vi "Clock Example.vi"() -> ()   [LabVIEW 2015]
uses:
  Forms/Rectangle/Rectangle.lvclass
  Image Editor Handler/Image Editor Handler.lvclass
  Forms/Shape/Shape.lvclass/Shape.ctl
  Forms/Rectangle/Rectangle.lvclass/Rectangle.ctl
  Forms/Shape/Write Color.vi
  Forms/Rectangle/Write Filled.vi
  Forms/Shape/Write Movable.vi
  Forms/Shape/Write Selectable.vi
  Forms/Shape/Shape.lvclass
  Forms/Link/Link.lvclass
panel:
  in  "2D Picture":picture
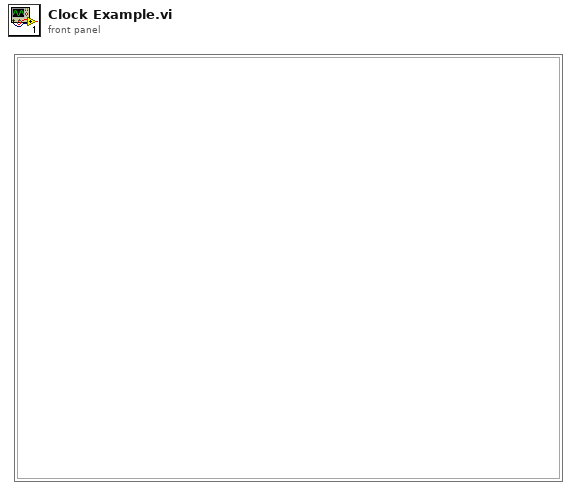
[diagram p1: front panel]
types:
  T1 = cluster{"Width":u16, "Style":enum32{"Solid", "Dash", "Dot", "DashDot", "DashDotDot"}}
  T2 = typedef "LVBoundsTypeDef.ctl" = cluster{"Width":u32, "Height":u32}
  T3 = cluster{"Rayon H":dbl, "Rayon M":dbl, "Rayon S":dbl}
  T4 = typedef "LVDateTimeRec.ctl" = cluster{"fractional second":dbl, "second":i32, "minute":i32, "hour":i32, "day of month":i32, "month":i32, "year":i32, "day of week":i32, "day of year":i32, "DST":i32}
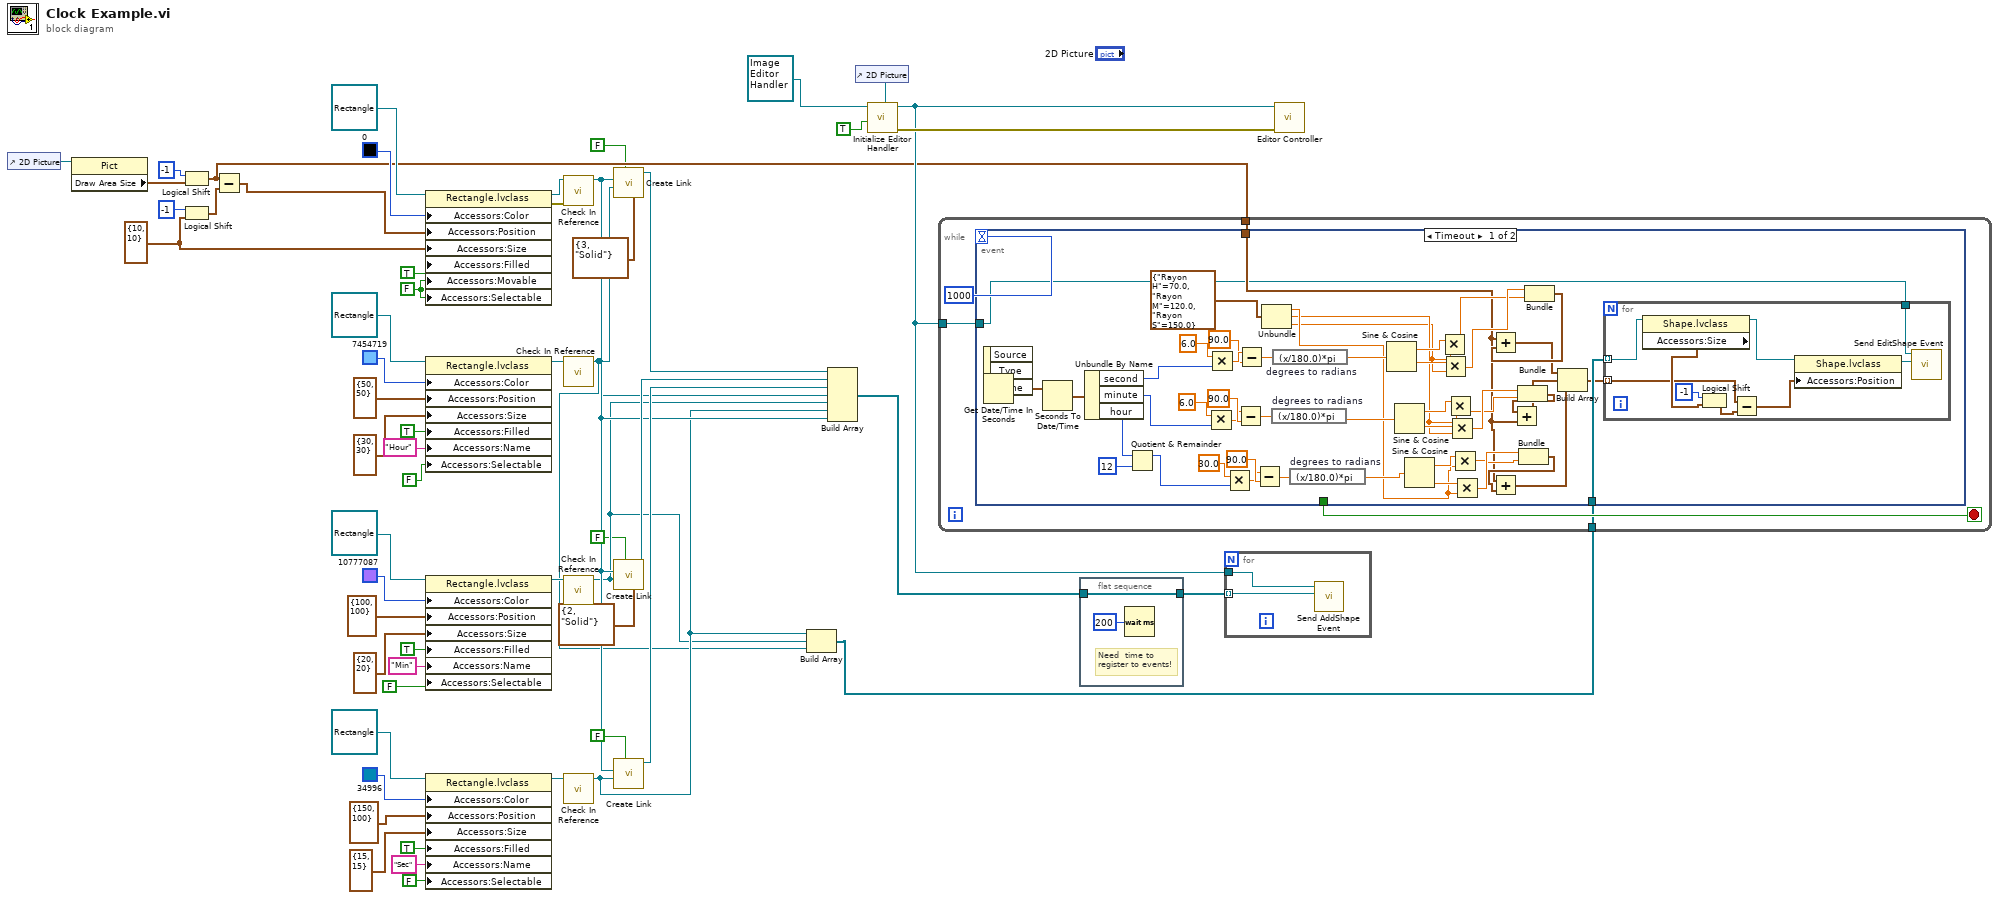
[diagram p0: block diagram]
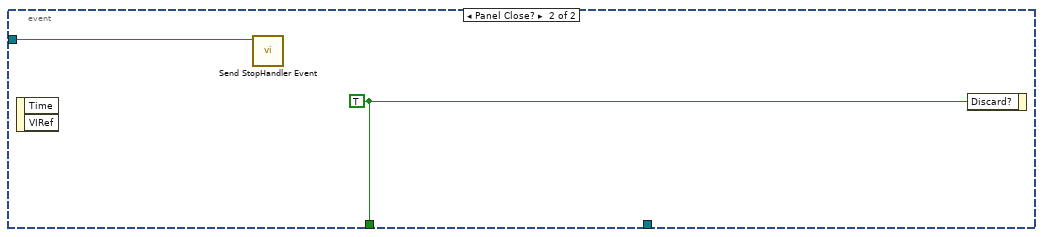
[diagram p2: hidden frame]
diagram:
  w39 = FALSE ("Movable")
  w19 = cluster{"Width":i32, "Height":i32} {"Width"=10, "Height"=10} ("Size")
  n1 = control-ref of="2D Picture"() -> (w27:refnum<vi>)
  n2 = property class="Pict"(reference=w27) -> ("Draw Area Size"=w25:T2)  [unwired: 1 in, 2 out]
  n3 = Logical Shift(y=i16 -1, x=w25) -> (x << y=w13:T2)
  n4 = Logical Shift(y=i16 -1, x=w19) -> (x << y=w23:cluster{"Width":i32, "Height":i32})
  n5 = Subtract(x=w13, y=w23) -> (x-y=w20:T2)
  n6 = property class="Rectangle.lvclass"(reference=refnum<class "Rectangle.lvclass"> refnum ("Rectangle.lvclass"), "Accessors:Color"=u32 0 ("Color"), "Accessors:Position"=w20, "Accessors:Size"=w19, "Accessors:Filled"=TRUE ("Filled"), "Accessors:Movable"=w39, "Accessors:Selectable"=w39) -> (reference out=w38:refnum<class "Rectangle.lvclass">, error out=w37:errorcluster)  [unwired: 1 in]
  n7 = property class="Rectangle.lvclass"(reference=refnum<class "Rectangle.lvclass"> refnum ("Rectangle.lvclass"), "Accessors:Color"=u32 7454719 ("Color"), "Accessors:Position"=cluster{"Left":i32, "Top":i32} {"Left"=50, "Top"=50} ("Position"), "Accessors:Size"=cluster{"Width":i32, "Height":i32} {"Width"=30, "Height"=30} ("Size"), "Accessors:Filled"=TRUE ("Filled"), "Accessors:Name"="Hour" ("Name"), "Accessors:Selectable"=FALSE ("Movable")) -> (reference out=w55:refnum<class "Rectangle.lvclass">)  [unwired: 1 in, 1 out]
  n8 = property class="Rectangle.lvclass"(reference=refnum<class "Rectangle.lvclass"> refnum ("Rectangle.lvclass"), "Accessors:Color"=u32 10777087 ("Color"), "Accessors:Position"=cluster{"Left":i32, "Top":i32} {"Left"=100, "Top"=100} ("Position"), "Accessors:Size"=cluster{"Width":i32, "Height":i32} {"Width"=20, "Height"=20} ("Size"), "Accessors:Filled"=TRUE ("Filled"), "Accessors:Name"="Min" ("Name"), "Accessors:Selectable"=FALSE ("Selectable")) -> (reference out=w50:refnum<class "Rectangle.lvclass">)  [unwired: 1 in, 1 out]
  n9 = property class="Rectangle.lvclass"(reference=refnum<class "Rectangle.lvclass"> refnum ("Rectangle.lvclass"), "Accessors:Color"=u32 34996 ("Color"), "Accessors:Position"=cluster{"Left":i32, "Top":i32} {"Left"=150, "Top"=100} ("Position"), "Accessors:Size"=cluster{"Width":i32, "Height":i32} {"Width"=15, "Height"=15} ("Size"), "Accessors:Filled"=TRUE ("Filled"), "Accessors:Name"="Sec" ("Name"), "Accessors:Selectable"=FALSE ("Selectable")) -> (reference out=w45:refnum<class "Rectangle.lvclass">)  [unwired: 1 in, 1 out]
  n10 = call "Check In Reference.vi"("error in (no error)"=w37, "Shape in"=w38) -> ("Shape Reference"=w18:refnum<data-value>)  [unwired: 8 in, 1 out]
  n11 = call "Check In Reference.vi"("Shape in"=w55) -> ("Shape Reference"=w15:refnum<data-value>)  [unwired: 9 in, 1 out]
  n12 = call "Check In Reference.vi"("Shape in"=w50) -> ("Shape Reference"=w16:refnum<data-value>)  [unwired: 9 in, 1 out]
  n13 = call "Check In Reference.vi"("Shape in"=w45) -> ("Shape Reference"=w17:refnum<data-value>)  [unwired: 9 in, 1 out]
  n14 = call "Create Link.vi"("Style"=T1 {"Width"=3, "Style"=enum."Solid"}, "Selectable"=FALSE, "Destination"=w15, "Source"=w18) -> ("Link Reference"=w36:refnum<data-value>)  [unwired: 6 in, 1 out]
  n15 = call "Create Link.vi"("Style"=T1 {"Width"=2, "Style"=enum."Solid"}, "Selectable"=FALSE, "Destination"=w16, "Source"=w18) -> ("Link Reference"=w35:refnum<data-value>)  [unwired: 6 in, 1 out]
  n16 = call "Create Link.vi"("Selectable"=FALSE, "Destination"=w17, "Source"=w18) -> ("Link Reference"=w34:refnum<data-value>)  [unwired: 7 in, 1 out]
  n17 = Build Array(w17, w16, w15) -> (w14:refnum<data-value>[])
  n18 = Build Array(w36, w35, w34, w15, w16, w17, w18) -> (w29:refnum<data-value>[])
  n19 = control-ref of="2D Picture"() -> (w31:refnum<vi>)
  n20 = call "Initialize Editor Handler.vi"("Clear Picture?"=TRUE ("Clean Picture?"), "PictureRef"=w31, "Editor Handler in"=refnum<class "Image Editor Handler.lvclass"> refnum) -> ("error out"=w33:errorcluster, "Editor Handler out"=w28:refnum<class "Image Editor Handler.lvclass">)  [unwired: 7 in]
  n21 = while {
    tunnel: w28 -> [w62]
    tunnel: w14 -> [w60]
    tunnel: w13 -> [w59]
    stop <- w63 stop-if-true
    n22 = event shown="[0] Timeout" {
      selector: _ -> [_ _]
      dyn-events: _ -> [_ _]
      timeout: 1000 -> [_ _]
      tunnel: [_ w122] -> w63
      tunnel: w62 -> [w71 w121]
      tunnel: w60 -> [w74 _]
      tunnel: w59 -> [w72 _]
      event Timeout {
        n23 = event-data() -> ()  [unwired: 1 in, 3 out]
        n24 = Get Date/Time In Seconds() -> (seconds since 1Jan1904=w111:timestamp)
        n25 = Seconds To Date/Time(time stamp (now)=w111) -> (date time rec=w110:T4)  [unwired: 1 in]
        n26 = Unbundle By Name(w110) -> ("second"=w96:i32, "minute"=w105:i32, "hour"=w70:i32)
        n27 = Quotient & Remainder(x=w70, y=12) -> (x-y*floor(x/y)=w68:i32)  [unwired: 1 out]
        n28 = Multiply(x=6.0, y=w105) -> (x*y=w107:dbl)
        n29 = Multiply(x=6.0, y=w96) -> (x*y=w103:dbl)
        n30 = Multiply(x=30.0, y=w68) -> (x*y=w98:dbl)
        n31 = Subtract(x=w107, y=90.0) -> (x-y=w106:dbl)
        n32 = Subtract(x=w103, y=90.0) -> (x-y=w104:dbl)
        n33 = Subtract(x=w98, y=90.0) -> (x-y=w97:dbl)
        n34 = Unbundle(T3 {"Rayon H"=70.0, "Rayon M"=120.0, "Rayon S"=150.0}) -> ("Rayon H"=w66:dbl, "Rayon M"=w65:dbl, "Rayon S"=w64:dbl)
        n35 = expression code="(x/180.0)*pi" "degrees to radians"(w106) -> (w93:dbl)
        n36 = expression code="(x/180.0)*pi" "degrees to radians"(w104) -> (w95:dbl)
        n37 = expression code="(x/180.0)*pi" "degrees to radians"(w97) -> (w94:dbl)
        n38 = Sine & Cosine(0:w95) -> (1:w87:dbl, 2:w88:dbl)
        n39 = Sine & Cosine(0:w93) -> (1:w89:dbl, 2:w92:dbl)
        n40 = Sine & Cosine(0:w94) -> (1:w90:dbl, 2:w91:dbl)
        n41 = Multiply(x=w87, y=w64) -> (x*y=w85:dbl)
        n42 = Multiply(x=w88, y=w64) -> (x*y=w86:dbl)
        n43 = Multiply(x=w89, y=w65) -> (x*y=w82:dbl)
        n44 = Multiply(x=w92, y=w65) -> (x*y=w83:dbl)
        n45 = Multiply(x=w90, y=w66) -> (x*y=w79:dbl)
        n46 = Multiply(x=w91, y=w66) -> (x*y=w80:dbl)
        n47 = Bundle(w83, w82) -> (w81:cluster{dbl, dbl})  [unwired: 1 in]
        n48 = Add(x=w81, y=w72) -> (x+y=w76:cluster{dbl, dbl})
        n49 = Bundle(w80, w79) -> (w78:cluster{dbl, dbl})  [unwired: 1 in]
        n50 = Add(x=w72, y=w78) -> (x+y=w75:cluster{dbl, dbl})
        n51 = Bundle(w86, w85) -> (w84:cluster{dbl, dbl})  [unwired: 1 in]
        n52 = Add(x=w72, y=w84) -> (x+y=w77:cluster{dbl, dbl})
        n53 = Build Array(w77, w76, w75) -> (w73:cluster{dbl, dbl}[])
        n54 = for {
          tunnel: w74 -> [w118] mode=indexing
          tunnel: w73 -> [w114] mode=indexing
          tunnel: w71 -> [w120]
          n55 = property class="Shape.lvclass"(reference=w118) -> (reference out=w117:refnum<data-value>, "Accessors:Size"=w115:cluster{"Width":i32, "Height":i32})  [unwired: 1 in, 1 out]
          n56 = Logical Shift(y=i16 -1, x=w115) -> (x << y=w113:cluster{"Width":i32, "Height":i32})
          n57 = Subtract(x=w114, y=w113) -> (x-y=w112:cluster{dbl, dbl})
          n58 = property class="Shape.lvclass"(reference=w117, "Accessors:Position"=w112) -> (reference out=w119:refnum<data-value>)  [unwired: 1 in, 1 out]
          n59 = call "Send EditShape Event.vi"("Shape"=w119, "Editor Handler in"=w120) -> ()  [unwired: 8 in, 2 out]
        }
      }
      event Panel Close? {
        w122 = TRUE ("Discard?")
        n60 = event-data() -> ()  [unwired: 1 in, 2 out]
        n61 = call "Send StopHandler Event.vi"("Editor Handler in"=w121) -> ()  [unwired: 9 in, 2 out]
        n62 = event-data("Discard?"=w122) -> ()  [unwired: 1 in, 1 out]
      }
    }
  }
  n63 = flat-sequence {
    tunnel: w29 -> [w123]
    tunnel: [w123] -> w30
    frame #0 {
      # "Need  time to register to events!"
      n64 = Wait (ms)(milliseconds to wait=u32 200) -> ()  [unwired: 1 out]
    }
  }
  n65 = for {
    tunnel: w30 -> [w125] mode=indexing
    tunnel: w28 -> [w126]
    n66 = call "Send AddShape Event.vi"("New Shape Reference"=w125, "Editor Handler in"=w126) -> ()  [unwired: 8 in, 2 out]
  }
  n67 = call "Editor Controller.vi"("error in (no error)"=w33, "Editor Handler in"=w28) -> ()  [unwired: 8 in, 2 out]
